vi "PrepareHWI.vi"(8 "error in (no error)":errorcluster, 9 "Master Device in":refnum<class "Master Device.lvclass">, 10 "Current Variables":T1[](array[typedef]), 11 "NI Card in":refnum<class "NI Card.lvclass">) -> (0 "error out":errorcluster, 2 "Master Device out":refnum<class "Master Device.lvclass">, 3 "NI Card out":refnum<class "NI Card.lvclass">)   [LabVIEW 2013, in "NI Card.lvclass"]
uses:
  NI Card.lvclass
  TypeDefs/Active procedure variables.ctl
  Master Device/Master Device.lvclass
  NI Card.lvclass/NI Card.ctl
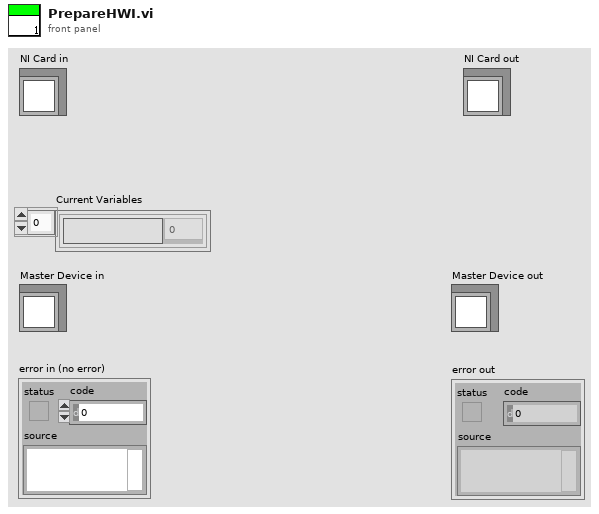
[diagram p1: front panel]
types:
  T1 = typedef "Active procedure variables.ctl" = cluster{"Procedure variable":string, "Value":dbl}
  T2 = cluster{"Triggering":bool[][], "Ramp Info":cluster{"Ramp Index":i32, "Ramp Time":dbl, "Number of Steps":i32}[], "VLIW Array":cluster{"Output Bits":u32, "Data Field":u32, "OP Code":u8, "Delay Count":u64}[]}
  T3 = cluster{"Ramp Index":i32, "Ramp Time":dbl, "Number of Steps":i32}[]
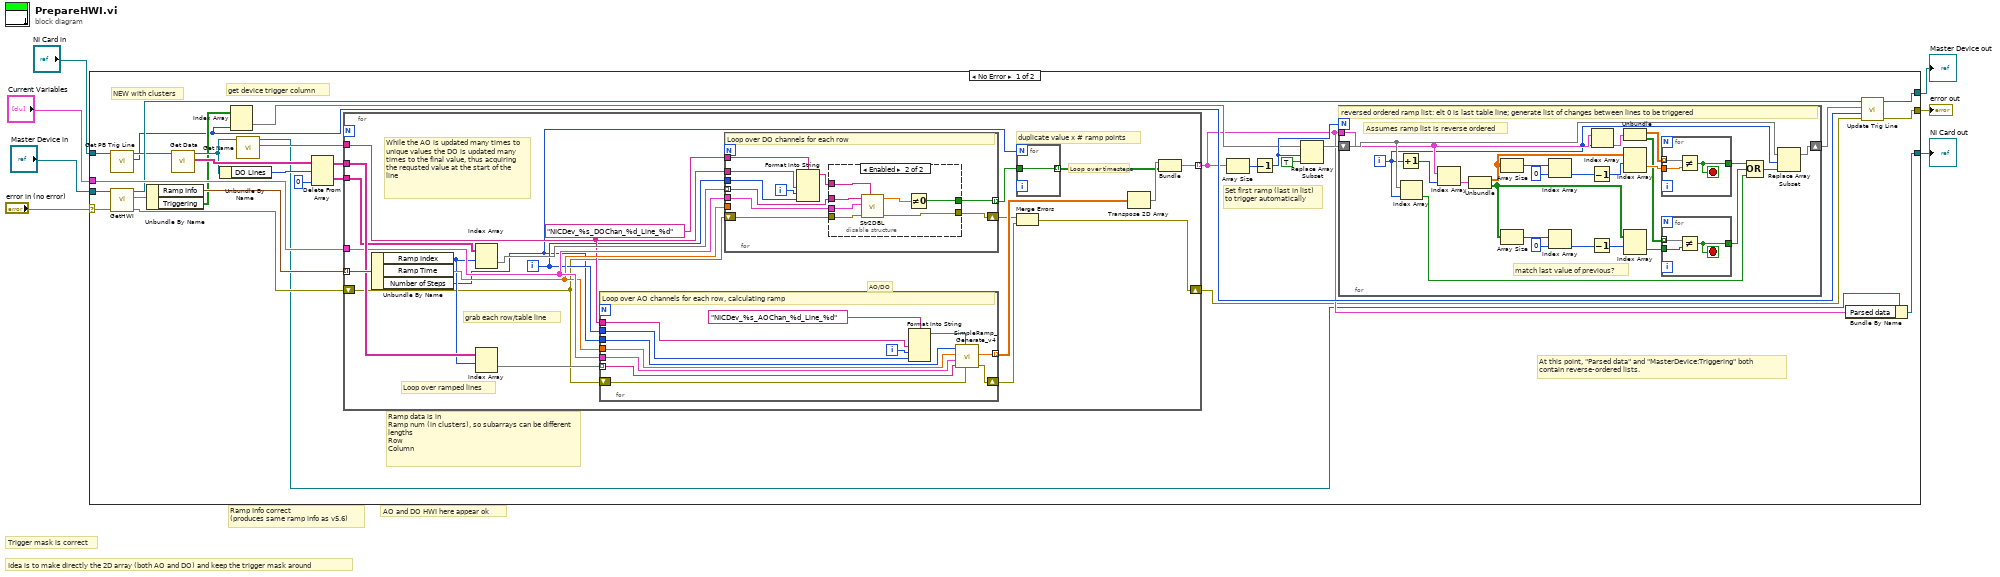
[diagram p0: block diagram]
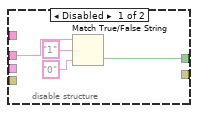
[diagram p2: hidden frame]
diagram:
  # "Idea is to make directly the 2D array (both AO and DO) and keep the trigger mask around"
  # "Trigger mask is correct"
  # "AO and DO HWI here appear ok"
  # "Ramp Info correct\n(produces same ramp info as v5.6)"
  n1 = case shown="No Error" "error in (no error)" {
    selector: "error in (no error)" -> [w36 w126]
    tunnel: [w33 w126] -> w6
    tunnel: [w31 w125] -> w4
    tunnel: "NI Card in" -> [w32 w125]
    tunnel: "Current Variables" -> [w35 _]
    tunnel: "Master Device in" -> [w37 w124]
    tunnel: [w34 w124] -> w1
    frame No Error {
      # "At this point, \"Parsed data\" and \"MasterDevice:Triggering\" both\ncontain reverse-ordered lists."
      # "get device trigger column"
      # "NEW with clusters"
      # "Set first ramp (last in list)\nto trigger automatically"
      # "Ramp data is in\nRamp num (in clusters), so subarrays can be different lengths\nRow\nColumn"
      n2 = call-dynamic "Get PB Trig Line.vi"("Device in"=w32) -> ("PB Trigger Line"=w12:u16, "Device out"=w16:refnum<class "NI Card.lvclass">)  [unwired: 8 in, 1 out]
      n3 = call-dynamic "GetHWI.vi"("error in (no error)"=w36, "Master Device in"=w37) -> ("error out"=w26:errorcluster, "Hardware Image"=w30:T2, "Master Device out"=w20:refnum<class "Master Device.lvclass">)  [unwired: 7 in]
      n4 = Unbundle By Name(w30) -> ("Ramp Info"=w28:T3, "Triggering"=w15:bool[][])
      n5 = call-dynamic "Get Data.vi"("Device in"=w16) -> ("Table Indicator"=w27:string[][], "Device out"=w24:refnum<class "NI Card.lvclass">)  [unwired: 7 in, 1 out]
      n6 = Unbundle By Name(w24) -> ("DO Lines"=w23:i32)
      n7 = Index Array(array=w15, index (col)=w12) -> (element=w14:bool[])  [unwired: 1 in]
      n8 = call-dynamic "Get Name.vi"("Device in"=w24) -> ("Name"=w29:string, "Device out"=w9:refnum<class "NI Card.lvclass">)  [unwired: 8 in, 1 out]
      n9 = Delete From Array(array=w27, length=w23, index (col)=0 ("disabled index (col)")) -> (deleted portion=w22:string[][], array with subset deleted=w25:string[][])  [unwired: 1 in]
      n10 = for {
        tunnel: w29 -> [w77]
        tunnel: w28 -> [w89] mode=indexing
        tunnel: w25 -> [w88]
        shift-right: [w74] -> w8
        shift-left: w26 -> [w75]
        tunnel: w35 -> [w85]
        tunnel: w22 -> [w83]
        tunnel: [w79] -> w10 mode=indexing
        i -> [w76]
        # "duplicate value x # ramp points"
        # "grab each row/table line"
        # "Loop over ramped lines"
        # "AO/DO"
        # "Loop over timesteps"
        # "While the AO is updated many times to unique values the DO is updated many times to the final value, thus acquiring the requsted value at the start of the line"
        n11 = Unbundle By Name(w89) -> ("Ramp Index"=w81:i32, "Ramp Time"=w84:dbl, "Number of Steps"=w71:i32)
        n12 = Index Array(array=w83, index (row)=w81) -> (element=w82:string[])  [unwired: 1 in]
        n13 = Index Array(array=w88, index (row)=w81) -> (element=w87:string[])  [unwired: 1 in]
        n14 = for {
          tunnel: [w123] -> w86 mode=indexing
          tunnel: w71 -> [w122]
          shift-right: [w121] -> w73
          shift-left: w75 -> [w120]
          tunnel: w77 -> [w119]
          tunnel: w87 -> [w117] mode=indexing
          tunnel: w85 -> [w116]
          tunnel: w84 -> [w115]
          tunnel: w76 -> [w113]
          i -> [w114]
          # "Loop over AO channels for each row, calculating ramp"
          n15 = Format Into String(format string="NICDev_%s_AOChan_%d_Line_%d", w119, w114, w113) -> (resulting string=w118:string)  [unwired: 2 in, 1 out]
          n16 = call "SimpleRamp_Generate_v4.vi"("error in (no error)"=w120, "Error Locator"=w118, "formula"=w117, "Current Variable settings"=w116, "dt"=w115, "Points"=w122) -> ("error out"=w121:errorcluster, "y values"=w123:dbl[])  [unwired: 2 out]
        }
        n17 = for {
          tunnel: w82 -> [w99] mode=indexing
          tunnel: w85 -> [w98]
          tunnel: w84 -> [_]
          tunnel: [w100] -> w72 mode=indexing
          shift-right: [w96] -> w69
          shift-left: w75 -> [w97]
          tunnel: "NICDev_%s_DOChan_%d_Line_%d" -> [w95]
          tunnel: w77 -> [w94]
          tunnel: w76 -> [w92]
          i -> [w93]
          # "Loop over DO channels for each row"
          n18 = Format Into String(format string=w95, w94, w93, w92) -> (resulting string=w91:string)  [unwired: 2 in, 1 out]
          n19 = disable-structure shown="Enabled" {
            disable-tunnel: [w104 w107] -> w100
            disable-tunnel: w99 -> [w103 w106]
            disable-tunnel: w98 -> [_ w110]
            disable-tunnel: w97 -> [_ w109]
            disable-tunnel: [_ w108] -> w96
            disable-tunnel: w91 -> [_ w105]
            frame Disabled {
              n20 = Match True/False String(2:"0" ("false string"), 3:"1" ("true string"), 4:w103) -> (0:w104:bool)  [unwired: 1 out]
            }
            frame Enabled {
              n21 = call "Str2DBL.vi"("Error Locator"=w105, "error in (no error)"=w109, "Current Variable settings"=w110, "formula"=w106) -> ("error out"=w108:errorcluster, "y value"=w111:dbl)  [unwired: 4 in]
              n22 = Not Equal To 0?(x=w111) -> (x != 0?=w107:bool)
            }
          }
        }
        n23 = for {
          N: w71 -> [_]
          tunnel: w72 -> [w90]
          tunnel: [w90] -> w70 mode=indexing
        }
        n24 = Merge Errors(w69, w73) -> (w74:errorcluster)
        n25 = Transpose 2D Array(2D array=w86) -> (transposed array=w80:dbl[][])
        n26 = Bundle(w80, w70) -> (w79:cluster{dbl[][], bool[][]})  [unwired: 1 in]
      }
      n27 = Array Size(array=w10) -> (size(s)=w11:i32)
      n28 = Decrement(x=w11) -> (x-1=w17:i32)
      n29 = Replace Array Subset(array=w14, new element=TRUE ("new element/subarray"), index=w17) -> (w21:bool[])
      n30 = for {
        N: w17 -> [_]
        tunnel: w10 -> [w48]
        shift-right: [w38] -> w13
        shift-left: w21 -> [w55]
        i -> [w45]
        # "match last value of previous?"
        # "Assumes ramp list is reverse ordered"
        # "reversed ordered ramp list: elt 0 is last table line; generate list of changes between lines to be triggered"
        n31 = Increment(x=w45) -> (x+1=w46:i32)
        n32 = Index Array(array=w55, index=w45) -> (element=w59:bool)
        n33 = Index Array(array=w48, index=w46) -> (element=w42:cluster{dbl[][], bool[][]})
        n34 = Unbundle(w42) -> (w41:dbl[][], w40:bool[][])
        n35 = Array Size(array=w41) -> (size(s)=w53:i32[])
        n36 = Array Size(array=w40) -> (size(s)=w62:i32[])
        n37 = Index Array(array=w53, index=0) -> (element=w50:i32)
        n38 = Index Array(array=w62, index=0) -> (element=w58:i32)
        n39 = Decrement(x=w50) -> (x-1=w49:i32)
        n40 = Decrement(x=w58) -> (x-1=w57:i32)
        n41 = Index Array(array=w48, index=w45) -> (element=w44:cluster{dbl[][], bool[][]})
        n42 = Unbundle(w44) -> (w43:dbl[][], w39:bool[][])
        n43 = Index Array(array=w41, index (row)=w49) -> (element=w51:dbl[])  [unwired: 1 in]
        n44 = Index Array(array=w40, index (row)=w57) -> (element=w60:bool[])  [unwired: 1 in]
        n45 = for {
          tunnel: w43 -> [w64] mode=indexing
          tunnel: w51 -> [w65]
          tunnel: [w63] -> w47
          stop <- w63 stop-if-true
          n46 = Not Equal?(x=w64, y=w65) -> (x != y?=w63:bool)
        }
        n47 = for {
          tunnel: w39 -> [w67] mode=indexing
          tunnel: w60 -> [w68]
          tunnel: [w66] -> w56
          stop <- w66 stop-if-true
          n48 = Not Equal?(x=w67, y=w68) -> (x != y?=w66:bool)
        }
        n49 = Compound Arithmetic op=OR(w47, w56, w59) -> (w54:bool)
        n50 = Replace Array Subset(array=w55, new element=w54, index=w45) -> (w38:bool[])
      }
      n51 = Bundle By Name(cluster=w9, "Parsed data"=w10) -> (w31:refnum<class "NI Card.lvclass">)
      n52 = call-dynamic "Update Trig Line.vi"("error in (no error)"=w8, "PB Trigger Line"=w12, "Triggering"=w13, "Master Device in"=w20) -> ("error out"=w33:errorcluster, "Master Device out"=w34:refnum<class "Master Device.lvclass">)  [unwired: 6 in]
    }
    frame Error {
    }
  }
  "error out" <- w6
  "NI Card out" <- w4
  "Master Device out" <- w1
